vi "Main User Console.vi"(8 "error in (no error)":errorcluster, 11 "Module_Refs":T2={"ModuleName"=enum."Controller", "Queue"=refnum, "user event"=refnum, "VI Refnum"=refnum, "ShowFP"=FALSE, "StatesTracking Enabled"=FALSE}) -> (0 "error out":errorcluster)   [LabVIEW 2019, in "UserConsole.lvlib"]
doc: "Main Module Template of the architecture. Use this as a template to integrate new independent processes into your application."
uses:
  UserConsole.lvlib
  Architecture/Typedefs/Enum_Module_Name.ctl
  Architecture/Architecture.lvlib
  Architecture/Typedefs/Message.ctl
  Architecture/Typedefs/Module References.ctl
  Typedefs/State Machine Data.ctl
  Architecture/Typedefs/Application Configuration.ctl
  Typedefs/Config.ctl
  Architecture/Modules/Module Template/SubVIs/Module Template Configuraton Extractor API.vi
  Architecture/Modules/Module Template/Typedefs/Config.ctl
  Architecture/Modules/Module Template/Module Template.lvlib
  Controller/Typedefs/State Machine States.ctl
  Controller/Controller.lvlib
panel:
  in  "User Console":T1
  in  "Stop App":bool
  out "Message":string
  in  "Stop Module":bool
  # "#Architecture\n\nPlace inside this box all visible data."
  # "USER CONSOLE"
  # "[Covers: SI1]"
  # "[Covers: UI1]"
  # "[Covers: UI2C]"
  # "[Covers: UI2]"
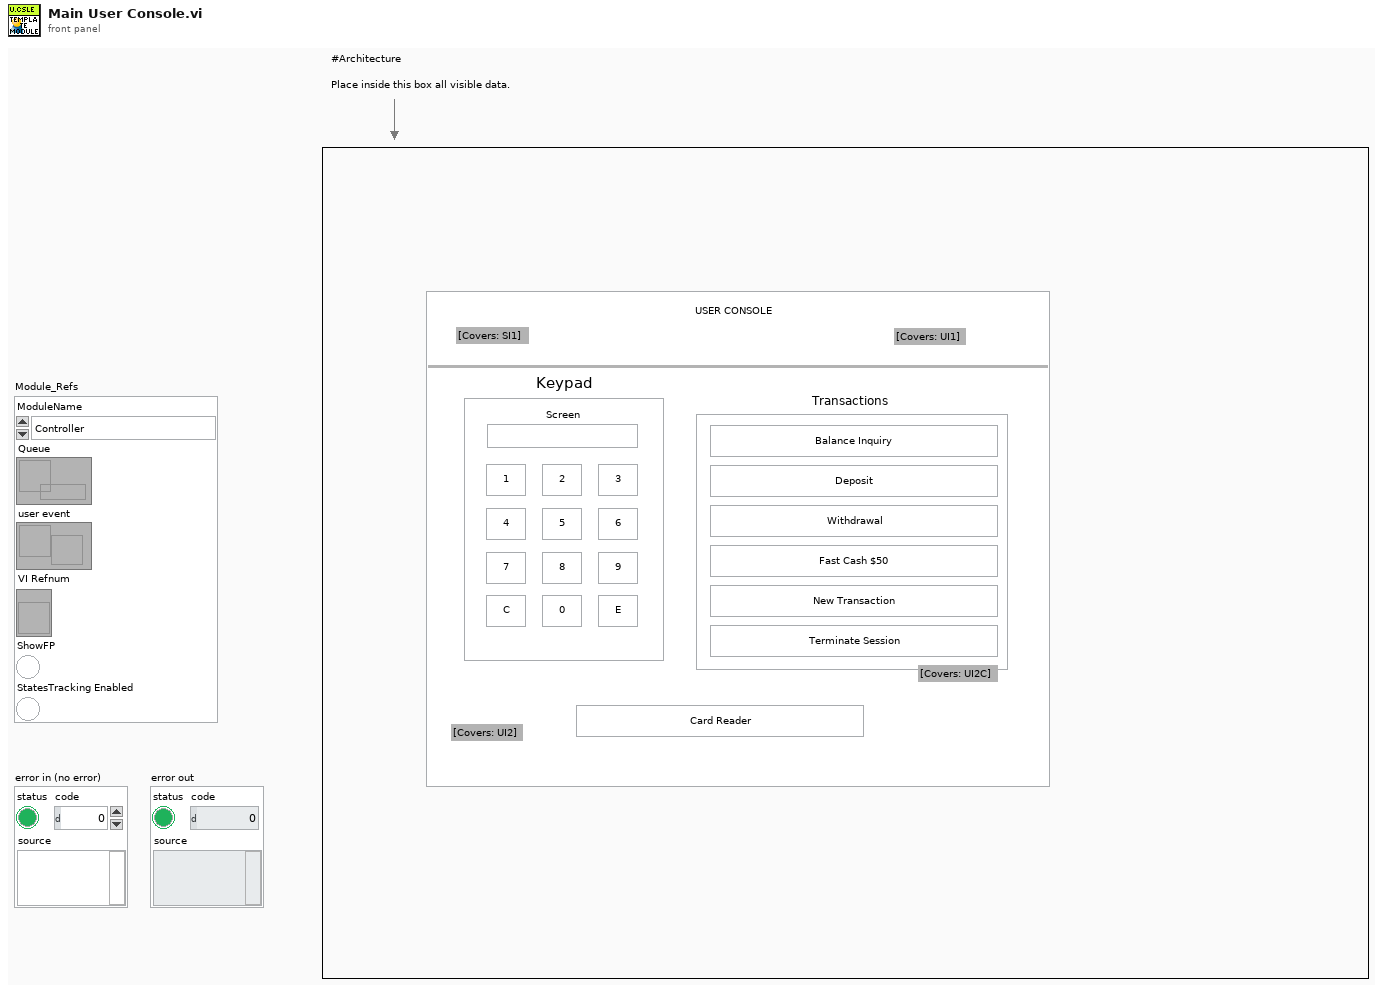
[diagram p1: front panel]
types:
  T1 = cluster{"Keypad":cluster{"Screen":string, "1":bool, "2":bool, "3":bool, "4":bool, "5":bool, "6":bool, "7":bool, "8":bool, "9":bool, "C":bool, "0":bool, "E":bool}, "Transactions":cluster{"Balance Inquiry":bool, "Deposit":bool, "Withdrawal":bool, "Fast Cash $50":bool, "New Transaction":bool, "Terminate Session":bool}, "Card Reader":bool}
  T2 = typedef "Architecture.lvlib/Module References.ctl" = cluster{"ModuleName":T3, "Queue":refnum<queue>, "user event":refnum<user-event>, "VI Refnum":refnum<vi>, "ShowFP":bool, "StatesTracking Enabled":bool}
  T3 = typedef "Architecture.lvlib/Enum_Module_Name.ctl" = enum16{"Configuration", "Error_Handler", "Log", "Database", "Controller", "User Console", "Display Console", "Sensor Interface"}
  T4 = typedef "UserConsole.lvlib/State Machine Data.ctl" = cluster{"Module_Refs":T2, "Response Data":variant, "Module Template Config":T5}
  T5 = typedef "UserConsole.lvlib/Config.ctl" = cluster{"Module Enabled":bool}
  T6 = enum32{"Invalid", "Standard", "Closed", "Hidden", "Minimized", "Maximized"}
  T7 = typedef "Controller.lvlib/State Machine States.ctl" = enum16{"Idle State", "Login State", "Balance Inquiry State", "Deposit State", "Withdrawal State", "Fast Cash State", "Terminate State", "Inactivity Timeout", "Wait For Transaction", "Add Balance"}
  T8 = typedef "Architecture.lvlib/Module Template.lvlib/Config.ctl" = cluster{"Module Enabled":bool}
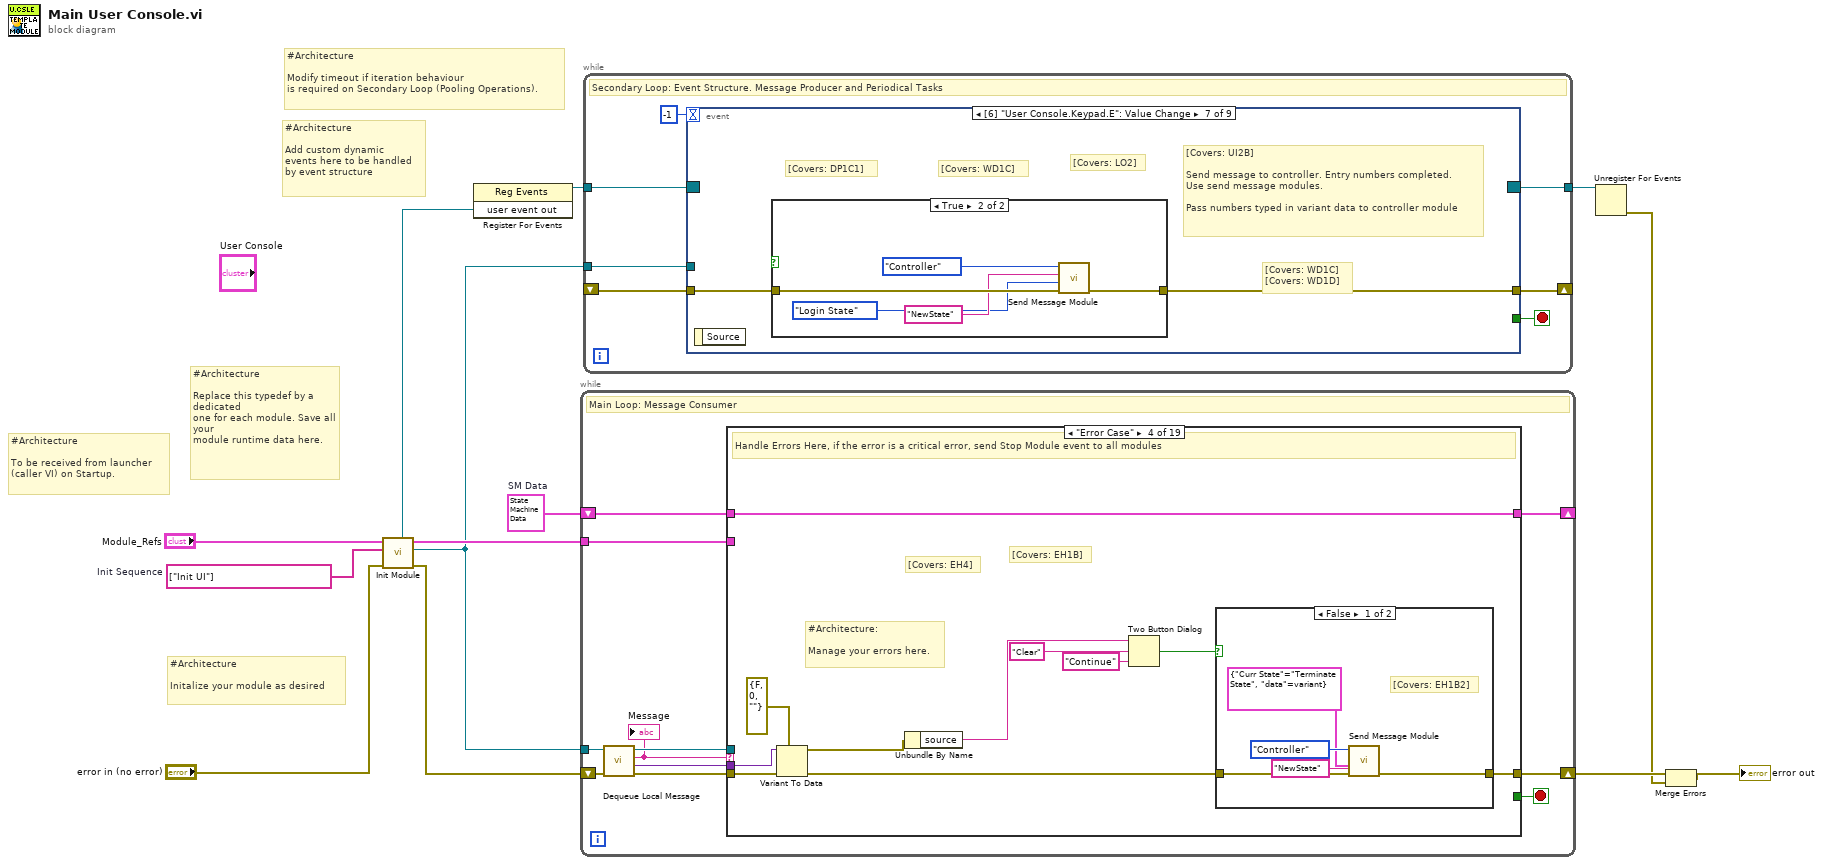
[diagram p0: block diagram]
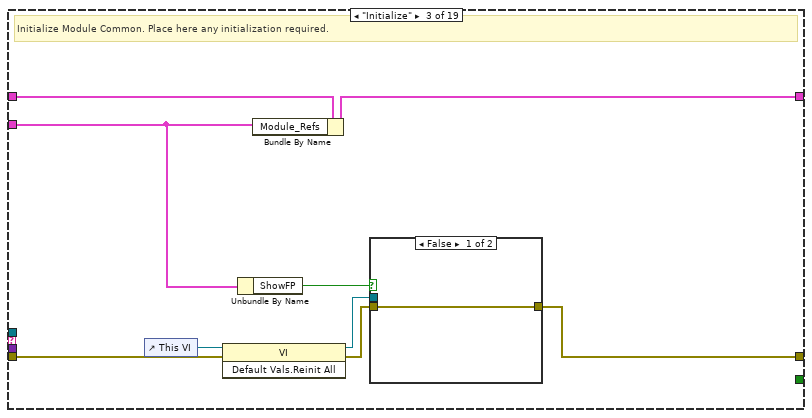
[diagram p4: hidden frame]
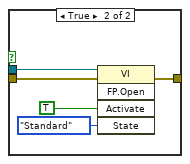
[diagram p5: hidden frame]
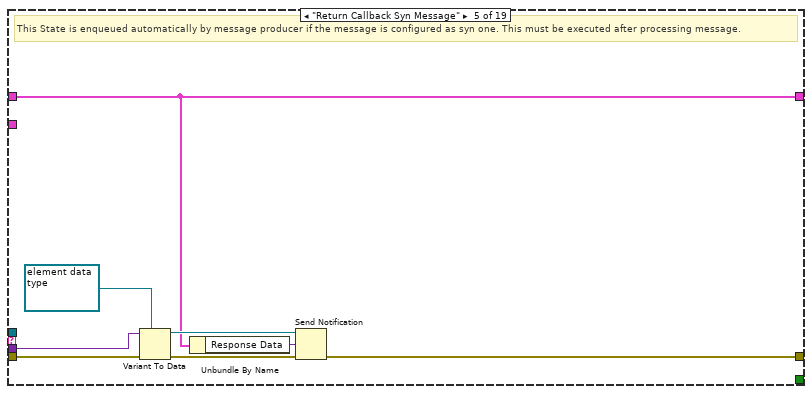
[diagram p7: hidden frame]
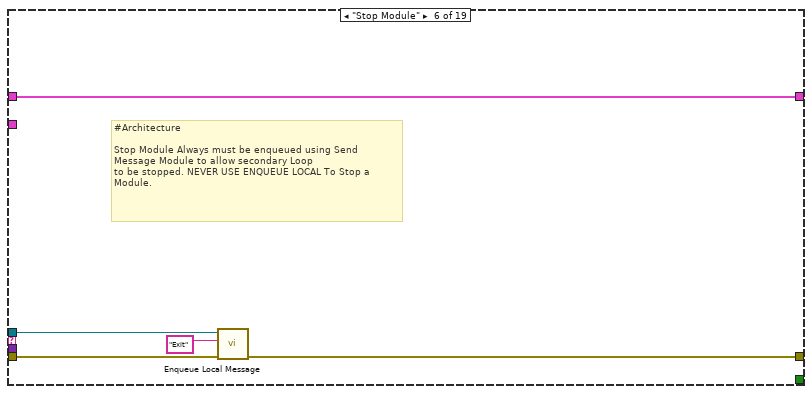
[diagram p8: hidden frame]
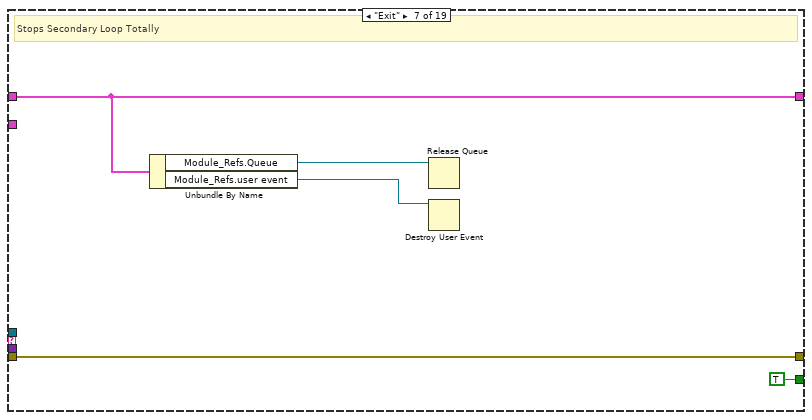
[diagram p9: hidden frame]
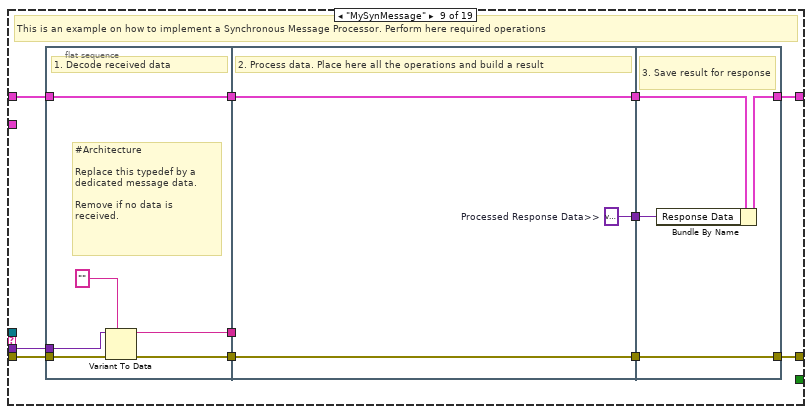
[diagram p11: hidden frame]
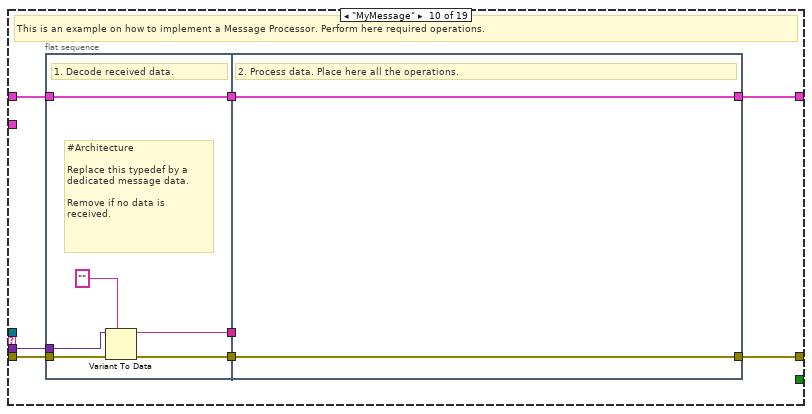
[diagram p12: hidden frame]
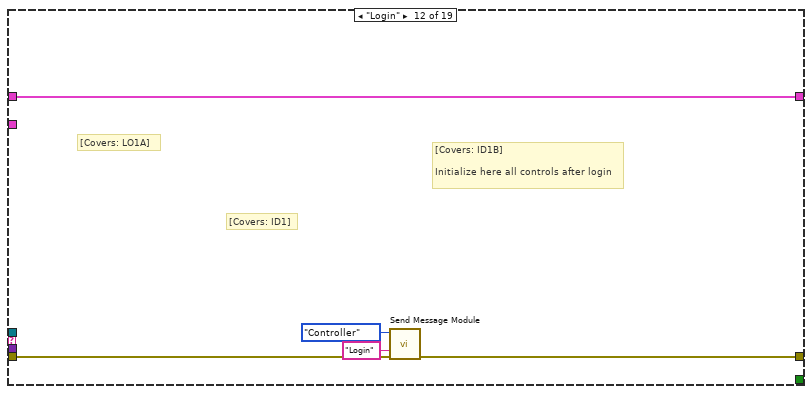
[diagram p14: hidden frame]
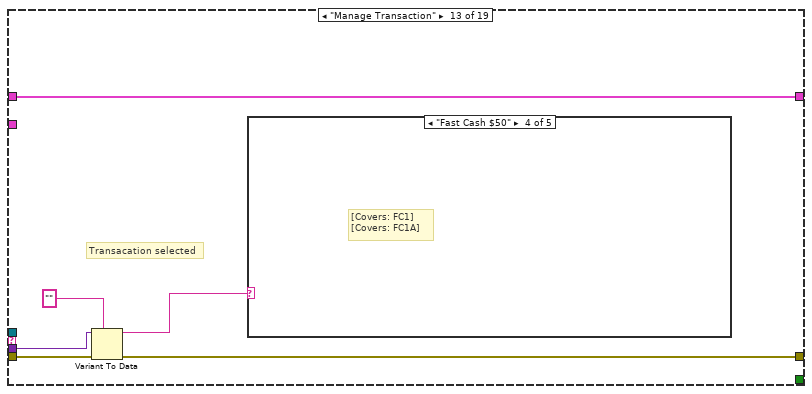
[diagram p15: hidden frame]
diagram:
  w10 = string[] ["Init UI"]  # Init Sequence
  w13 = T4 {"Module_Refs"={"ModuleName"=enum."Controller", "Queue"=refnum, "user event"=refnum, "VI Refnum"=refnum, "ShowFP"=FALSE, "StatesTracking Enabled"=FALSE}, "Response Data"=variant, "Module Template Config"={"Module Enabled"=FALSE}}  # SM Data
  # "#Architecture\n\nModify timeout if iteration behaviour \nis required on Secondary Loop (Pooling Operations)."
  # "#Architecture\n\nAdd custom dynamic \nevents here to be handled \nby event structure"
  # "#Architecture\n\nInitalize your module as desired"
  # "#Architecture\n\nTo be received from launcher \n(caller VI) on Startup."
  # "#Architecture\n\nReplace this typedef by a dedicated \none for each module. Save all your \nmodule runtime data here."
  n1 = call "Init Module.vi"("error in (no error)"="error in (no error)", "Init Sequence"=w10, "Module Refs"="Module_Refs") -> ("error out"=w12:errorcluster, "queue out"=w1:refnum<queue>, "Module Refs Out"=w3:T2, "user event out"=w2:refnum<user-event>)  [unwired: 5 in]
  n2 = register-events(w2) -> (reference out=w9:refnum<event-registration>)  [unwired: 2 in, 1 out]
  n3 = while {
    shift-right: [w23] -> _
    shift-left: w13 -> [w24]
    shift-right: [w22] -> w7
    shift-left: w12 -> [w20]
    tunnel: w1 -> [w21]
    tunnel: w3 -> [w14]
    stop <- w15 stop-if-true
    # "Main Loop: Message Consumer"
    n4 = call "Dequeue Local Message.vi"("error in"=w20, "Msg queue in"=w21) -> ("error out"=w19:errorcluster, "Data"=w16:variant, "Message"=w17:string, "queue out"=w18:refnum<queue>)  [unwired: 6 in]
    "Message" <- w17
    n5 = case shown="\"Error Case\"" w17 {
      selector: w17 -> [_ _ _ _ _ _ _ _ _ _ _ _ _ _ w136 _ _ _ w168]
      tunnel: w24 -> [w26 w28 w37 w54 w62 w73 w76 w80 w91 w112 w122 w127 w133 w135 w143 w148 w157 w159 w173]
      tunnel: [w26 w28 w35 w54 w62 w73 w76 w80 w90 w105 w122 w127 w133 w135 w143 w148 w150 w159 w173] -> w23
      tunnel: w19 -> [w25 w27 w36 w53 w68 w72 w78 w79 w84 w108 w121 w126 w132 w134 w140 w147 w156 w158 w172]
      tunnel: [w25 w27 w31 w46 w67 w71 w78 w79 w89 w111 w121 w125 w131 w134 w137 w146 w151 w158 w162] -> w22
      tunnel: w18 -> [_ _ _ _ _ w70 _ _ _ _ _ _ _ _ w138 w145 _ _ w169]
      tunnel: w16 -> [_ _ _ w52 w65 _ _ _ w83 w107 _ _ w130 _ w139 _ w155 _ w170]
      tunnel: [_ _ _ _ _ _ TRUE _ _ _ _ _ _ _ _ _ _ _ _] -> w15
      tunnel: w14 -> [_ _ w34 _ _ _ _ _ _ _ _ _ _ _ _ _ _ _ _]
      frame "--------State Machine Arquitechture Operations--------" {
      }
      frame "Idle", Default {
        # "Use this state to make iterations if required."
      }
      frame "Initialize" {
        # "Initialize Module Common. Place here any initialization required."
        n6 = control-ref of="This VI"() -> (w29:refnum<vi>)
        n7 = invoke class="VI" method="Default Vals.Reinit All"(reference=w29, error in=w36) -> (reference out=w32:refnum<vi>, error out=w33:errorcluster)  [unwired: 1 in, 1 out]
        n8 = Unbundle By Name(w34) -> ("ShowFP"=w30:bool)
        n9 = Bundle By Name(cluster=w37, "Module_Refs"=w34) -> (w35:T4)
        n10 = case shown="False" w30 {
          tunnel: w33 -> [w38 w43]
          tunnel: [w38 w42] -> w31
          tunnel: w32 -> [_ w41]
          frame False {
          }
          frame True {
            n11 = invoke class="VI" method="FP.Open"(reference=w41, error in=w43, "Activate"=TRUE ("Activate?"), "State"=T6."Standard") -> (error out=w42:errorcluster)  [unwired: 1 in, 4 out]
          }
        }
      }
      frame "Error Case" {
        # "[Covers: EH4]"
        # "[Covers: EH1B]"
        # "#Architecture: \n\nManage your errors here."
        # "Handle Errors Here, if the error is a critical error, send Stop Module event to all modules"
        n12 = Variant To Data(error in=w53, type=errorcluster {"status"=FALSE, "code"=0, "source"=""} ("error constant"), Variant=w52) -> (data=w50:errorcluster, error out=w47:errorcluster)
        n13 = Unbundle By Name(w50) -> ("source"=w49:string)
        n14 = Two Button Dialog(message=w49, 1:"Continue" ("F button name (\"Cancel\")"), 2:"Clear" ("T button name (\"OK\")")) -> (T button?=w44:bool)
        n15 = case shown="False" w44 {
          tunnel: w47 -> [w59 w60]
          tunnel: [w58 w60] -> w46
          frame False {
            # "[Covers: EH1B2]"
            n16 = call "Send Message Module.vi"("Error In"=w59, "Data"=cluster{"Curr State":T7, "data":variant} {"Curr State"=enum."Terminate State", "data"=variant} ("data"), "Message"="NewState", "Target ModuleName In"=Enum_Module_Name."Controller") -> ("error in (no error)"=w58:errorcluster)  [unwired: 7 in]
          }
          frame True {
            # "[Covers: EH1B1]"
          }
        }
      }
      frame "Return Callback Syn Message" {
        # "This State is enqueued automatically by message producer if the message is configured as syn one. This must be executed after processing message."
        n17 = Variant To Data(error in=w68, type=refnum<notifier> refnum ("notifier out"), Variant=w65) -> (data=w63:refnum<notifier>, error out=w66:errorcluster)
        n18 = Unbundle By Name(w62) -> ("Response Data"=w61:variant)
        n19 = Send Notification(notification=w61, notifier=w63, error in (no error)=w66) -> (error out=w67:errorcluster)  [unwired: 1 out]
      }
      frame "Stop Module" {
        # "#Architecture\n\nStop Module Always must be enqueued using Send Message Module to allow secondary Loop\nto be stopped. NEVER USE ENQUEUE LOCAL To Stop a Module."
        n20 = call "Enqueue Local Message.vi"("error in"=w72, "Message"="Exit", "Msg queue in"=w70) -> ("error out"=w71:errorcluster)  [unwired: 7 in, 1 out]
      }
      frame "Exit" {
        # "Stops Secondary Loop Totally"
        n21 = Unbundle By Name(w76) -> ("Module_Refs.Queue"=w75:refnum<queue>, "Module_Refs.user event"=w74:refnum<user-event>)
        n22 = Release Queue(queue=w75) -> ()  [unwired: 2 in, 3 out]
        n23 = Destroy User Event(user event=w74) -> ()  [unwired: 1 in, 1 out]
      }
      frame "--------------State Machine Custom States-------------" {
      }
      frame "MySynMessage" {
        # "This is an example on how to implement a Synchronous Message Processor. Perform here required operations"
        n24 = flat-sequence {
          tunnel: w84 -> [w95]
          tunnel: w91 -> [w97]
          tunnel: [w97] -> w88
          tunnel: [w93] -> w87
          tunnel: w83 -> [w94]
          tunnel: [w92] -> w82
          tunnel: w88 -> [w100]
          tunnel: w87 -> [w99]
          tunnel: [w100] -> w86
          tunnel: [w99] -> w85
          tunnel: w82 -> [_]
          tunnel: [w98] -> w81
          tunnel: [w103] -> w89
          tunnel: [w102] -> w90
          tunnel: w86 -> [w104]
          tunnel: w85 -> [w103]
          tunnel: w81 -> [w101]
          frame #0 {
            # "#Architecture\n\nReplace this typedef by a dedicated message data.\n\nRemove if no data is received."
            # "1. Decode received data"
            n25 = Variant To Data(error in=w95, type="", Variant=w94) -> (data=w92:string, error out=w93:errorcluster)
          }
          frame #1 {
            w98 = variant  # Processed Response Data>>
            # "2. Process data. Place here all the operations and build a result"
          }
          frame #2 {
            # "3. Save result for response"
            n26 = Bundle By Name(cluster=w104, "Response Data"=w101) -> (w102:T4)
          }
        }
      }
      frame "MyMessage" {
        # "This is an example on how to implement a Message Processor. Perform here required operations."
        n27 = flat-sequence {
          tunnel: w108 -> [w116]
          tunnel: w112 -> [w118]
          tunnel: [w118] -> w110
          tunnel: [w114] -> w109
          tunnel: w107 -> [w115]
          tunnel: [w113] -> w106
          tunnel: w110 -> [w119]
          tunnel: w109 -> [w120]
          tunnel: w106 -> [_]
          tunnel: [w120] -> w111
          tunnel: [w119] -> w105
          frame #0 {
            # "#Architecture\n\nReplace this typedef by a dedicated message data.\n\nRemove if no data is received."
            # "1. Decode received data."
            n28 = Variant To Data(error in=w116, type="", Variant=w115) -> (data=w113:string, error out=w114:errorcluster)
          }
          frame #1 {
            # "2. Process data. Place here all the operations."
          }
        }
      }
      frame "Init UI" {
        # "[Covers: IS1]\n\nPlace here all calls to property nodes to \ninitialize UI controls and Indicators.\n\n• Card Reader control is enabled.\n• Keypad control is disabled.\n• All Transactions are disabled."
      }
      frame "Login" {
        # "[Covers: LO1A]"
        # "[Covers: ID1B]\n\nInitialize here all controls after login"
        # "[Covers: ID1]"
        n29 = call "Send Message Module.vi"("Error In"=w126, "Message"="Login", "Target ModuleName In"=Enum_Module_Name."Controller") -> ("error in (no error)"=w125:errorcluster)  [unwired: 8 in]
      }
      frame "Manage Transaction" {
        # "Transacation selected"
        n30 = Variant To Data(error in=w132, type="", Variant=w130) -> (data=w128:string, error out=w131:errorcluster)
        n31 = case shown="\"Fast Cash $50\"" w128 {
          frame "Balance Inquiry" {
            # "[Covers: BI1] \n[Covers: BI1A] \n[Covers: BI1B]"
            # "[Covers: BI1]"
          }
          frame "Deposit" {
            # "[Covers: DP1C] \n[Covers: DP1C1] \n[Covers: DP1C2] \n[Covers: DP1C3]"
            # "[Covers: DP1A]"
          }
          frame "Withdrawal" {
            # "[Covers: WD1C] \n[Covers: WD1D]"
            # "[Covers: WD1] \n[Covers: WD1A]"
          }
          frame "Fast Cash $50" {
            # "[Covers: FC1] \n[Covers: FC1A]"
          }
          frame ? {
            # "[Covers: FC1] \n[Covers: FC1A]"
          }
        }
      }
      frame "--------------Dynamic Events Messages----------------" {
      }
      frame "Message: MyMessage" {
        n32 = Match Pattern(string=w136, regular expression="Message: ") -> (after substring=w141:string)  [unwired: 1 in, 3 out]
        n33 = call "Enqueue Local Message.vi"("error in"=w140, "Data"=w139, "Message"=w141, "Msg queue in"=w138) -> ("error out"=w137:errorcluster)  [unwired: 6 in, 1 out]
      }
      frame "Message: Stop Module" {
        n34 = call "Enqueue Local Message.vi"("error in"=w147, "Message"="Stop Module", "Msg queue in"=w145) -> ("error out"=w146:errorcluster)  [unwired: 7 in, 1 out]
      }
      frame "Message: Load Config" {
        # "Get dedicated data for this module from \ngeneral DVR configuration and save it into \nSM Data to use it on runtime."
        # "Message used to receive configuration from a configuration module. Decode dedicated typedef and save it into SM Data"
        n35 = Variant To Data(error in=w156, type=refnum<data-value> refnum ("data value reference"), Variant=w155) -> (data=w153:refnum<data-value>, error out=w152:errorcluster)
        n36 = call-poly "Read Configuration API.vi"("error constant"=w152, "General Config DVR In"=w153) -> ("error out"=w151:errorcluster, "Module Template Config"=w149:T8)  [unwired: 8 in]
        n37 = Bundle By Name(cluster=w157, "Module Template Config"=w149) -> (w150:T4)
      }
      frame "------------Synchronous Event Messages--------------" {
      }
      frame "SynMessage: MySynMessage" {
        # "Use this case as a handler for Synchronous messages. This state queues a message for the desired"
        n38 = call "Extract Synchronous Data.vi"("error in 2"=w172, "Variant"=w170) -> ("error in"=w171:errorcluster, "Data Out"=w165:variant, "notifier out"=w160:refnum<notifier>)  [unwired: 7 in]
        n39 = Match Pattern(string=w168, regular expression="SynMessage: ") -> (after substring=w166:string)  [unwired: 1 in, 3 out]
        n40 = call "Enqueue Local Message.vi"("error in"=w171, "Data"=w165, "Message"=w166, "Msg queue in"=w169) -> ("error out"=w164:errorcluster, "queue out"=w163:refnum<queue>)  [unwired: 6 in]
        n41 = call "Enqueue Local Message.vi"("error in"=w164, "Data"=w160, "Message"="Return Callback Syn Message", "Msg queue in"=w163) -> ("error out"=w162:errorcluster)  [unwired: 6 in, 1 out]
      }
    }
  }
  n42 = while {
    tunnel: w9 -> [w180]
    tunnel: w1 -> [w177]
    tunnel: [w176] -> w8
    shift-right: [w174] -> _
    shift-left: _ -> [w175]
    stop <- w178 stop-if-true
    # "Secondary Loop: Event Structure. Message Producer and Periodical Tasks"
    n43 = event shown="[6] \"User Console.Keypad.E\": Value Change" {
      selector: w180 -> [_ _ _ _ _ _ _ _ _]
      dyn-events: [_ _ _ _ _ _ _ _ _] -> w176
      timeout: -1 -> [_ _ _ _ _ _ _ _ _]
      tunnel: [FALSE w189 TRUE _ _ _ _ _ _] -> w178
      tunnel: w177 -> [_ w194 w196 _ w205 _ _ _ w219]
      tunnel: w175 -> [w181 w193 w199 w201 w207 w208 w210 w218 w225]
      tunnel: [w181 w192 w197 w200 w206 w208 w209 w217 w224] -> w174
      event Timeout {
        n44 = event-data() -> ()  [unwired: 1 in, 1 out]
      }
      event User Event {
        # "Send message to local queue. \n(Message Consumer)"
        # "Processes an external event and enqueues a message to the local queue. It can be synchronous (with response) or NOT."
        n45 = event-data() -> ("syn"=w186:bool, "Message"=w188:string, "Data"=w191:variant)  [unwired: 1 in]
        n46 = Select(t="SynMessage: " ("string"), s=w186, f="Message: " ("string")) -> (s? t:f=w183:string)
        n47 = Concatenate Strings(w183, w188) -> (w190:string)
        n48 = call "Enqueue Local Message.vi"("error in"=w193, "Data"=w191, "Message"=w190, "Msg queue in"=w194) -> ("error out"=w192:errorcluster)  [unwired: 6 in, 1 out]
        n49 = Equal?(x=w188, y="Stop Module") -> (x = y?=w189:bool)
      }
      event "Stop Module": Value Change {
        n50 = event-data() -> ()  [unwired: 1 in, 1 out]
        n51 = call "Enqueue Local Message.vi"("error in"=w199, "Message"="Stop Module", "Msg queue in"=w196) -> ("error out"=w197:errorcluster)  [unwired: 7 in, 1 out]
      }
      event "Stop App": Value Change {
        w203 = TRUE  # All Modules
        # "Send Stop To All Modules"
        n52 = event-data() -> ()  [unwired: 1 in, 1 out]
        n53 = call "Send Message Modules.vi"("All Modules"=w203, "Error In"=w201, "Message"="Stop Module") -> ("error in (no error)"=w200:errorcluster)  [unwired: 8 in]
      }
      event "User Console.Card Reader": Value Change {
        # "[Covers: LO1]"
        # "[Covers: UI2A]\n\nQueue local message to handle the event of card insertion"
        n54 = event-data() -> ()  [unwired: 1 in, 1 out]
        n55 = call "Enqueue Local Message.vi"("error in"=w207, "Message"="Login", "Msg queue in"=w205) -> ("error out"=w206:errorcluster)  [unwired: 7 in, 1 out]
      }
      event "User Console.Keypad.C": Value Change {
        # "[Covers: UI2B]\n\nClear any entered numbers in the keypad"
        n56 = event-data() -> ()  [unwired: 1 in, 1 out]
      }
      event "User Console.Keypad.E": Value Change {
        # "[Covers: WD1C] \n[Covers: WD1D]"
        # "[Covers: WD1C]"
        # "[Covers: DP1C1]"
        # "[Covers: LO2]"
        # "[Covers: UI2B]\n\nSend message to controller. Entry numbers completed. \nUse send message modules. \n\nPass numbers typed in variant data to controller module"
        n57 = event-data() -> ()  [unwired: 1 in, 1 out]
        n58 = case shown="True" {
          selector: _ -> [_ _]
          tunnel: w210 -> [_ w214]
          tunnel: [_ w213] -> w209
          frame False {
          }
          frame True {
            n59 = call "Send Message Module.vi"("Error In"=w214, "Data"=State_Machine_States."Login State" ("Curr State"), "Message"="NewState", "Target ModuleName In"=Enum_Module_Name."Controller") -> ("error in (no error)"=w213:errorcluster)  [unwired: 7 in]
          }
        }
      }
      event "User Console.Keypad.1", "User Console.Keypad.2", "User Console.Keypad.3", "User Console.Keypad.4", "User Console.Keypad.5", "User Console.Keypad.6", "User Console.Keypad.7", "User Console.Keypad.8", "User Console.Keypad.9", "User Console.Keypad.0": Value Change {
        w216 = ""  # Typed text
        # "[Covers: UI2B]\n\nShow typed numbers into Keypad Screen"
        n60 = event-data() -> ()  [unwired: 1 in, 1 out]
        n61 = property on="Screen" class="Str"(error in=w218, "Value"=w216) -> (error out=w217:errorcluster)  [unwired: 1 in, 1 out]
      }
      event "User Console.Transactions.Balance Inquiry", "User Console.Transactions.Deposit", "User Console.Transactions.Withdrawal", "User Console.Transactions.Fast Cash $50", "User Console.Transactions.New Transaction", "User Console.Transactions.Terminate Session": Value Change {
        # "[Covers: UI2C]\n\nQueue local message to manage transaction selected. \n\nPass selected transaction to message consumer"
        n62 = event-data() -> ("CtlRef"=w223:refnum<vi>)  [unwired: 1 in]
        n63 = property class="Bool"(reference=w223) -> ("Label.Text"=w222:string)  [unwired: 1 in, 2 out]
        n64 = To Variant(anything=w222) -> (Variant=w221:variant)
        n65 = call "Enqueue Local Message.vi"("error in"=w225, "Data"=w221, "Message"="Manage Transaction", "Msg queue in"=w219) -> ("error out"=w224:errorcluster)  [unwired: 6 in, 1 out]
      }
    }
  }
  n66 = Unregister For Events(event registration refnum=w8) -> (error out=w6:errorcluster)  [unwired: 1 in]
  n67 = Merge Errors(w7, w6) -> (→"error out":errorcluster)
